vi "SS2 Live_Save HDF5 8-bit Gate Image.vi"(6 "Compression":bool, 7 "Replace?":bool, 8 "error in (no error)":errorcluster, 9 "Image Name":string, 10 "Data":u8[][](array[numeric]), 11 "ref in":T1 format="%.0x") -> (0 "error out":errorcluster, 3 "ref out":T1 format="%.0x")   [LabVIEW 2019]
uses:
  <vilib>/addons/h5labview2/base/hid_t.ctl
  <vilib>/addons/h5labview2/base/lib_path.vi
  <vilib>/addons/h5labview2/base/H5Equery.vi
  <vilib>/addons/h5labview2/dataset/H5Dwrite.llb/H5Dwrite.xnode
  <vilib>/addons/h5labview2/props/H5P.lvlib
  <vilib>/addons/h5labview2/space/H5S.lvlib
  <vilib>/addons/h5labview2/type/H5T.lvlib
  <vilib>/addons/h5labview2/dataset/H5D.lvlib
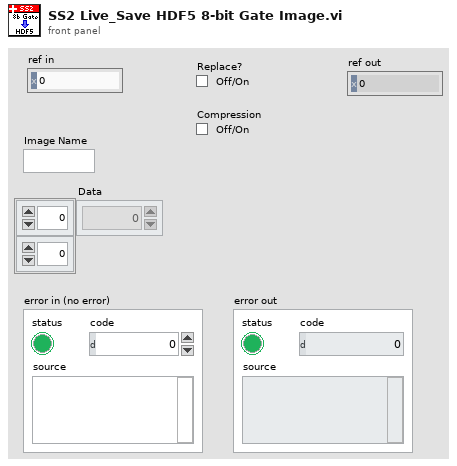
[diagram p1: front panel]
types:
  T1 = typedef "hid_t.ctl" = i32
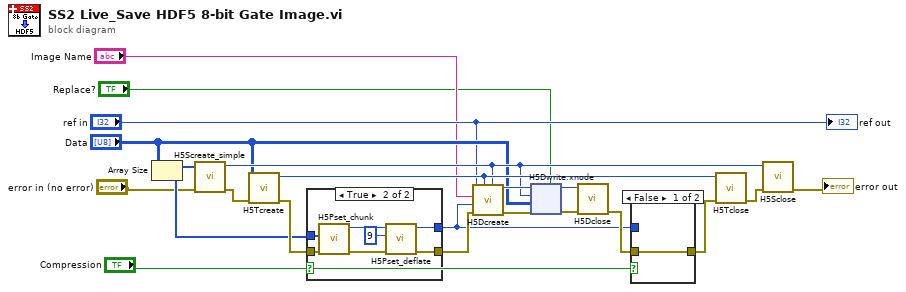
[diagram p0: block diagram]
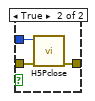
[diagram p2: hidden frame]
diagram:
  n1 = Array Size(array="Data") -> (size(s)=w9:i32[])
  n2 = call <vilib>:"H5Screate_simple.vi"("error in (no error)"="error in (no error)", "dims"=w9) -> ("error out"=w17:errorcluster, "space out"=w11:T1)  [unwired: 7 in, 1 out]
  n3 = call <vilib>:"H5Tcreate.vi"("error in (no error)"=w17, "type variant"="Data") -> ("error out"=w16:errorcluster, "type out"=w13:i32)  [unwired: 7 in, 1 out]
  n4 = case shown="True" "Compression" {
    tunnel: w16 -> [w22 w29]
    tunnel: [_ w28] -> w1
    tunnel: [w22 w24] -> w10
    tunnel: w9 -> [_ w23]
    frame False {
    }
    frame True {
      n5 = call <vilib>:"H5Pset_chunk.vi"("error in (no error)"=w29, "chunk size"=w23) -> ("error out"=w26:errorcluster, "prop out"=w27:T1)  [unwired: 8 in]
      n6 = call <vilib>:"H5Pset_deflate.vi"("error in (no error)"=w26, "level"=u8 9, "prop in"=w27) -> ("error out"=w24:errorcluster, "prop out"=w28:T1)  [unwired: 7 in]
    }
  }
  n7 = call <vilib>:"H5Dcreate.vi"("space id"=w11, "type id"=w13, "error in (no error)"=w10, "props id"=w1, "name"="Image Name", "loc in"="ref in") -> ("error out"=w15:errorcluster, "dset out"=w18:T1)  [unwired: 2 in]
  n8 = xnode "H5Dwrite.xnode"("replace? (F)"="Replace?", "error in (no error)"=w15, "data"="Data", "file space"=w11, "ref in"=w18) -> ("error out"=w21:errorcluster, "ref out"=w19:i32)  [unwired: 2 in, 1 out]
  n9 = call <vilib>:"H5Dclose.vi"("error in (no error)"=w21, "dset in"=w19) -> ("error out"=w20:errorcluster)  [unwired: 9 in]
  n10 = case shown="False" "Compression" {
    tunnel: w20 -> [w30 w33]
    tunnel: [w30 w32] -> w14
    tunnel: w1 -> [_ w31]
    frame False {
    }
    frame True {
      n11 = call <vilib>:"H5Pclose.vi"("error in (no error)"=w33, "props in"=w31) -> ("error out"=w32:errorcluster)  [unwired: 9 in]
    }
  }
  n12 = call <vilib>:"H5Tclose.vi"("error in (no error)"=w14, "type in"=w13) -> ("error out"=w12:errorcluster)  [unwired: 9 in]
  n13 = call <vilib>:"H5Sclose.vi"("error in (no error)"=w12, "space in"=w11) -> ("error out"=→"error out":errorcluster)  [unwired: 9 in]
  "ref out" <- "ref in"
